vi "open config file.vi"(8 "error in (no error)":errorcluster, 10 "create file if necessary (T)":bool=TRUE, 11 "file name":string) -> (0 "error out":errorcluster, 2 "file created?":bool, 3 "Refnum out":T1)   [LabVIEW 2024, in "API Config Files.lvlib"]
doc: "This function opens a configuration .ini file for reading or writing, given the file name as a string input. Internally, it uses the Application Directory.vi that returns the app directory, and build the full path for the configuration file. The function returns a Refnum to the opened configuration file."
uses:
  API Config Files.lvlib
  <vilib>/Utility/config.llb/Config Data RefNum.ctl
  <vilib>/Utility/config.llb/NI_LVConfig.lvlib
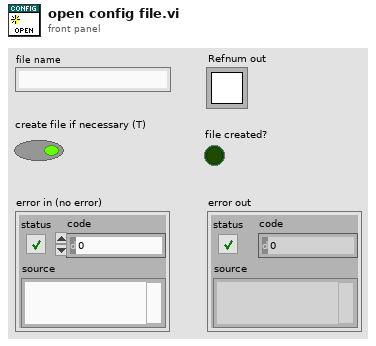
[diagram p1: front panel]
types:
  T1 = typedef "NI_LVConfig.lvlib/Config Data RefNum.ctl" = refnum<k1>
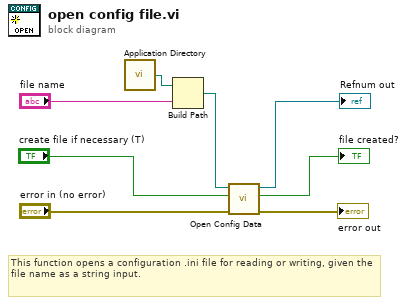
[diagram p0: block diagram]
diagram:
  # "This function opens a configuration .ini file for reading or writing, given the file name as a string input."
  n1 = call <vilib>:"Application Directory.vi"() -> ("Application Directory"=w7:path)
  n2 = Build Path(base path=w7, name or relative path="file name") -> (appended path=w5:path)
  n3 = call <vilib>:"Open Config Data.vi"("error in (no error)"="error in (no error)", "create file if necessary (T)"="create file if necessary (T)", "configuration file path"=w5) -> ("error out"=→"error out":errorcluster, "file created?"=→"file created?":bool, "refnum"=→"Refnum out":T1)  [unwired: 6 in]
